vi "Read GroupName.vi"(8 "error in (no error)":errorcluster, 11 "VariableGroup in":refnum<class "VariableGroup.lvclass">) -> (0 "error out":errorcluster, 2 "GroupName":string, 3 "VariableGroup out":refnum<class "VariableGroup.lvclass">)   [LabVIEW 2013, in "VariableGroup.lvclass"]
uses:
  VariableGroup.lvclass
  VariableGroup.lvclass/VariableGroup.ctl
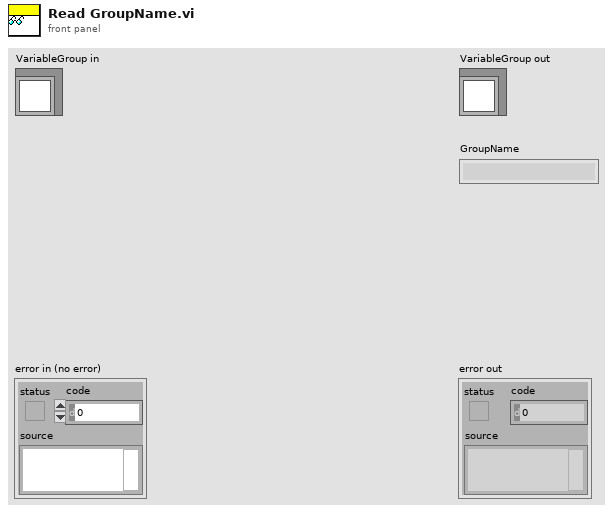
[diagram p1: front panel]
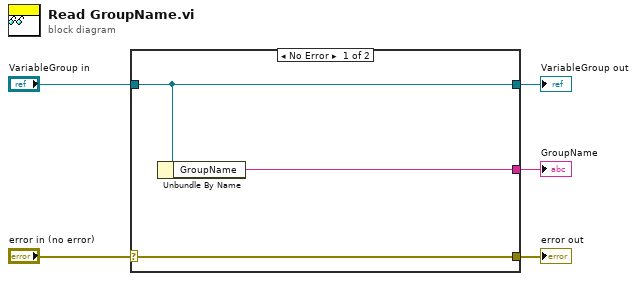
[diagram p0: block diagram]
diagram:
  n1 = case shown="No Error" "error in (no error)" {
    selector: "error in (no error)" -> [w8 w9]
    tunnel: [w8 w9] -> w4
    tunnel: [w7 w10] -> w2
    tunnel: "VariableGroup in" -> [w7 w10]
    tunnel: [w6 _] -> w1
    frame No Error {
      n2 = Unbundle By Name(w7) -> ("GroupName"=w6:string)
    }
    frame Error {
    }
  }
  "error out" <- w4
  "VariableGroup out" <- w2
  "GroupName" <- w1
